vi "serial getattr.vi"(8 "error in (no error)":errorcluster, 11 "portHandle in":i32) -> (0 "error out":errorcluster, 2 "options":string, 3 "portHandle out":i32)   [LabVIEW 2016, in "navX Library.lvlib"]
uses:
  navX Library.lvlib
  libc.so.6
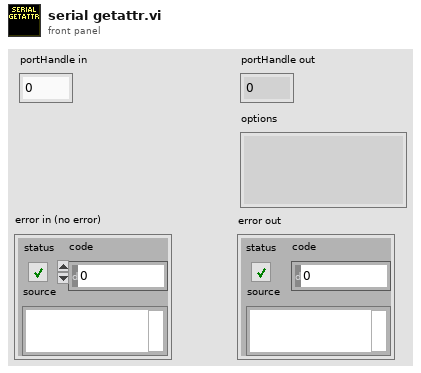
[diagram p1: front panel]
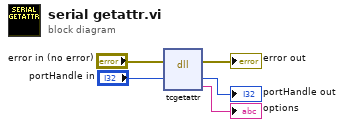
[diagram p0: block diagram]
diagram:
  n1 = dll-call lib="libc.so.6" fn="tcgetattr"(error in="error in (no error)", "portHandle"="portHandle in") -> (error out=→"error out":errorcluster, "portHandle"=→"portHandle out":i32, "options"=→"options":string)  [unwired: 4 in, 1 out]
